vi "Gray Demo.vi"() -> ()   [LabVIEW 2012, in "Picture Box Tools.lvlib"]
uses:
  Picture Box Tools.lvlib
  <vilib>/picture/picture.llb/imagedata.ctl
panel:
  in  "阙值":u8=128
  out "2 Value":picture
  in  "image data":T1={"image type"=0, "image depth"=24, "image"=array[50850 elements], "mask"=[], "colors"=[], "Rectangle"={"left"=0, "top"=0, "right"=150, "bottom"=113}} caption="图像数据"
  out "Gray Image":picture
  out "RGB Image":picture
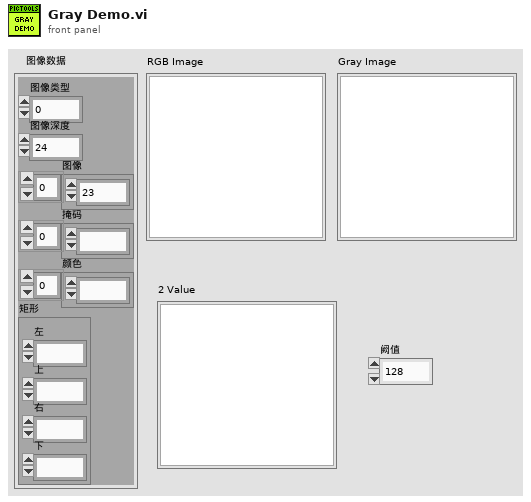
[diagram p1: front panel]
types:
  T1 = typedef "imagedata.ctl" = cluster{"image type":i32, "image depth":i32, "image":u8[], "mask":u8[], "colors":u32[], "Rectangle":cluster{"left":i16, "top":i16, "right":i16, "bottom":i16}}
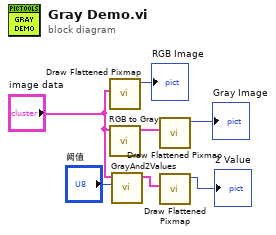
[diagram p0: block diagram]
diagram:
  n1 = call <vilib>:"Draw Flattened Pixmap.vi"("image data"="image data") -> ("new picture"=→"RGB Image":picture)  [unwired: 8 in]
  n2 = call "RGB to Gray.vi"("image data"="image data") -> ("输出簇"=w7:T1)  [unwired: 9 in, 1 out]
  n3 = call "GrayAnd2Values.vi"("阙值"="阙值", "image data"="image data") -> ("输出簇"=w3:T1)  [unwired: 8 in, 1 out]
  n4 = call <vilib>:"Draw Flattened Pixmap.vi"("image data"=w7) -> ("new picture"=→"Gray Image":picture)  [unwired: 8 in]
  n5 = call <vilib>:"Draw Flattened Pixmap.vi"("image data"=w3) -> ("new picture"=→"2 Value":picture)  [unwired: 8 in]
